vi "Analog Waveform DAQ Engine.vi"(8 "error in":errorcluster, 10 "DAQ Engine":refnum<notifier>, 11 "Sequence Context In":refnum<k7>) -> (0 "error out":errorcluster)   [LabVIEW 2023, in "LTT_TeststandSteptypes.lvlib"]
uses:
  LTT_TeststandSteptypes.lvlib
  HardwareAbstractionLayer_LVOOP/Main/Class Ref.ctl
  HardwareAbstractionLayer_LVOOP/DMM/DMM.lvclass
  HardwareAbstractionLayer_LVOOP/Function Generator/Function Generator.lvclass
  HardwareAbstractionLayer_LVOOP/Oscilloscope/Oscilloscope.lvclass
  HardwareAbstractionLayer_LVOOP/PowerSupply/PowerSupply.lvclass
  HardwareAbstractionLayer_LVOOP/Teststand/Teststand.lvclass
  HardwareAbstractionLayer_LVOOP/Analog Output/AO/AO.lvclass
  HardwareAbstractionLayer_LVOOP/Analog Input/AI/AI.lvclass
  HardwareAbstractionLayer_LVOOP/Database/Database.lvclass
  HardwareAbstractionLayer_LVOOP/Digital Output/DO_class/DO.lvclass
  HardwareAbstractionLayer_LVOOP/Digital Input/DI_class/DI.lvclass
  HardwareAbstractionLayer_LVOOP/PWM Output/PWM Output_class/PWM Output.lvclass
  HardwareAbstractionLayer_LVOOP/PWM Input/PWM Input_class/PWM Input.lvclass
  HardwareAbstractionLayer_LVOOP/NI Switch/NISwitch_class/NISwitch.lvclass
  HardwareAbstractionLayer_LVOOP/Modbus/Modbus_class/Modbus.lvclass
  HardwareAbstractionLayer_LVOOP/CAN/CAN Lib/CAN_class/CAN.lvclass
  HardwareAbstractionLayer_LVOOP/Main/Class Options.ctl
  <vilib>/Utility/error.llb/DialogType.ctl
  HardwareAbstractionLayer_LVOOP/Main/Main.lvclass
panel:
  in  "stop":bool
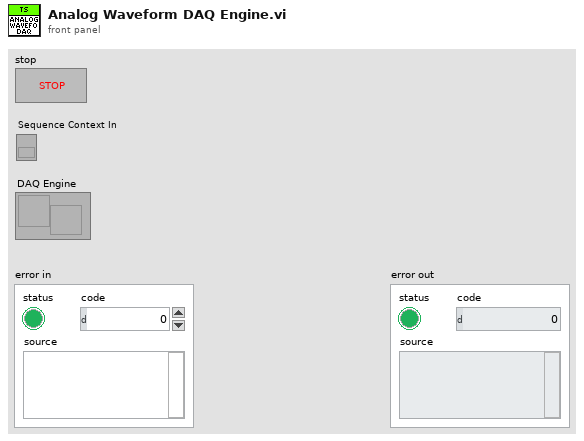
[diagram p1: front panel]
types:
  T1 = typedef "HardwareAbstractionLayer_LVOOP.lvlib/Main.lvclass/Class Ref.ctl" = cluster{"DMM":refnum<class "DMM.lvclass">, "Function Generator":refnum<class "Function Generator.lvclass">, "Oscilloscope":refnum<class "Oscilloscope.lvclass">, "PowerSupply":refnum<class "PowerSupply.lvclass">, "Teststand":refnum<class "Teststand.lvclass">, "AO":refnum<class "AO.lvclass">, "AI":refnum<class "AI.lvclass">, "Database":refnum<class "Database.lvclass">, "AO Waveform Generation":refnum<class "AO.lvclass">, "DO":refnum<class "DO.lvclass">, "DI":refnum<class "DI.lvclass">, "PWM Output":refnum<class "PWM Output.lvclass">, "PWM Input":refnum<class "PWM Input.lvclass">, "RelayOutput":refnum<class "NISwitch.lvclass">, "Modbus":refnum<class "Modbus.lvclass">, "CAN":refnum<class "CAN.lvclass">}
  T2 = typedef "HardwareAbstractionLayer_LVOOP.lvlib/Main.lvclass/Class Options.ctl" = enum16{"Init All Class", "Read All Class", "Write AI Class", "Write AO Class", "Write AO Waveform Generation", "Write DI Class", "Write DO Class", "Write PWM Input Class", "Write PWM Output Class", "Exit"}
  T3 = typedef "DialogType.ctl" = u16
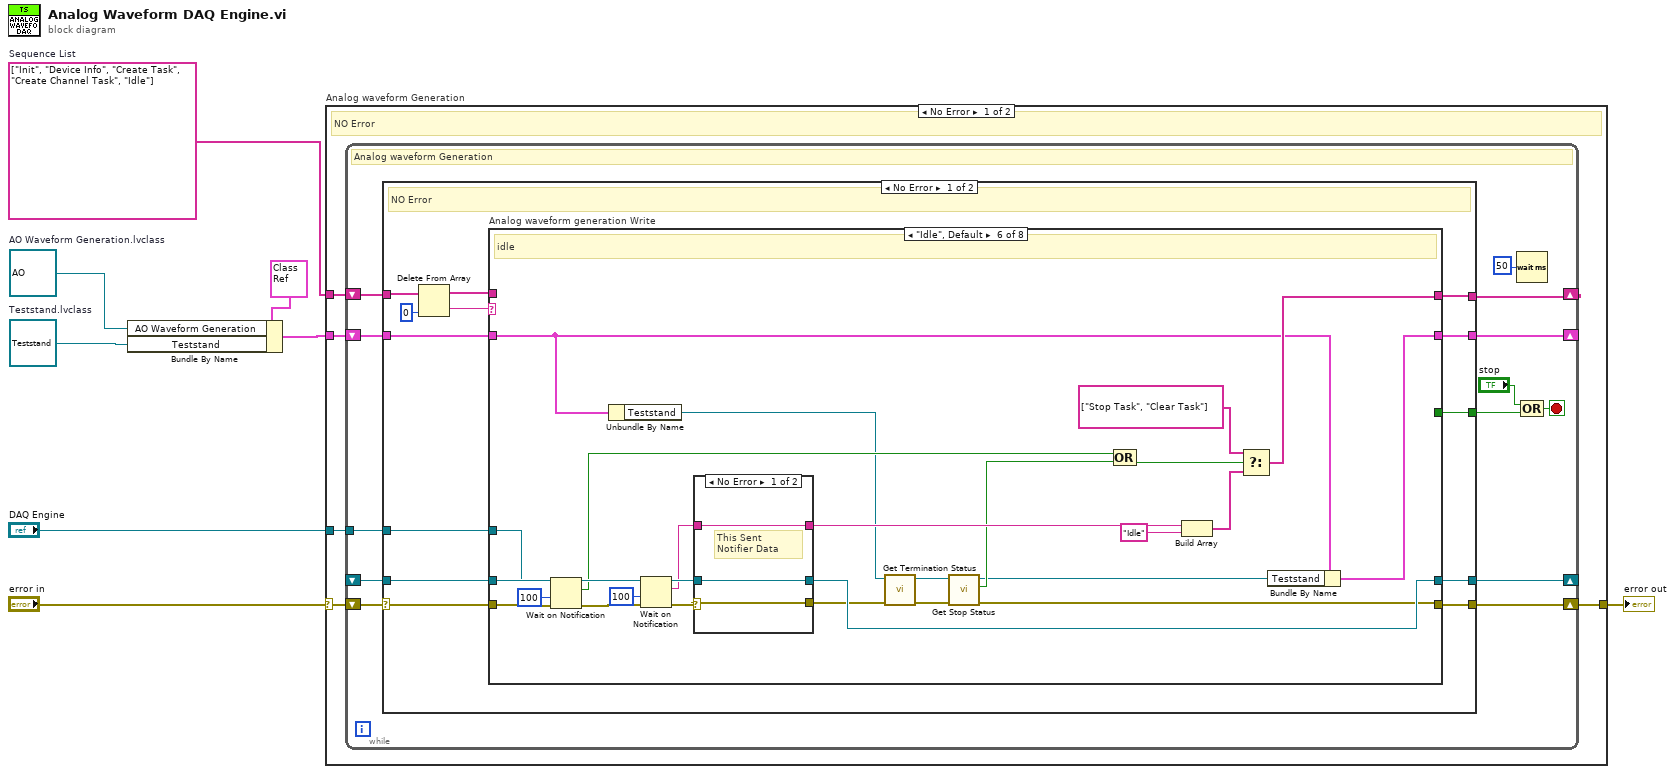
[diagram p0: block diagram]
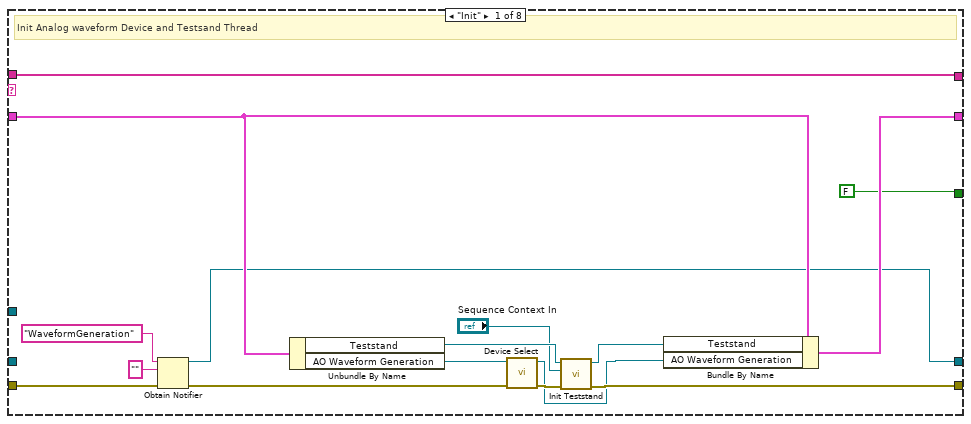
[diagram p2: hidden frame]
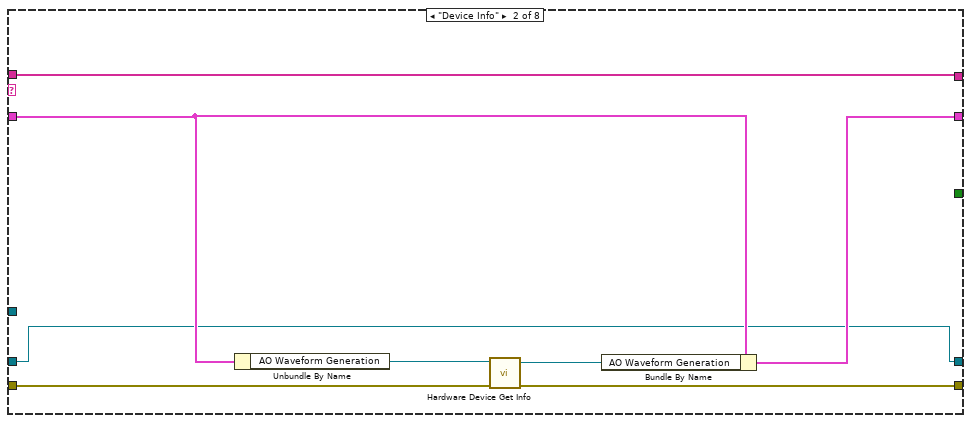
[diagram p3: hidden frame]
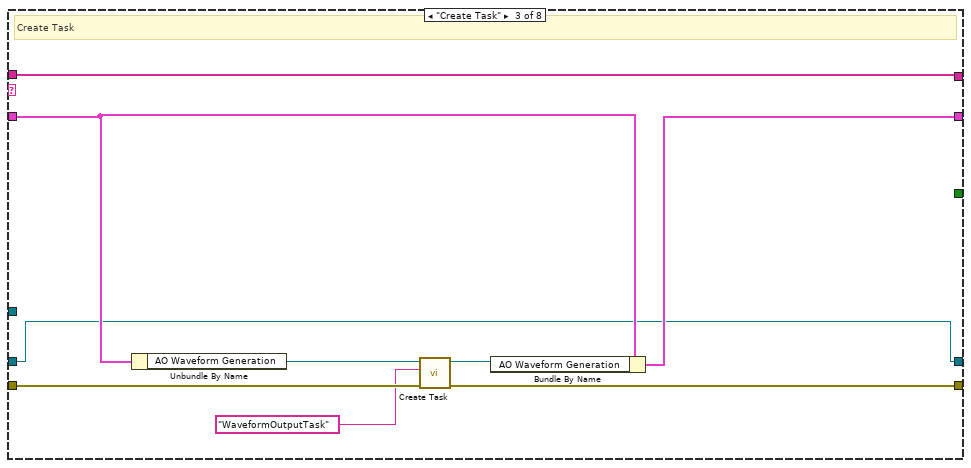
[diagram p4: hidden frame]
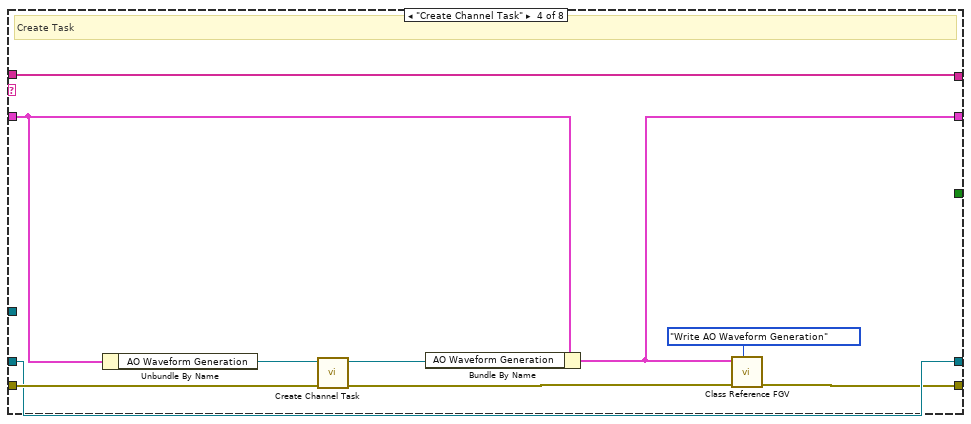
[diagram p5: hidden frame]
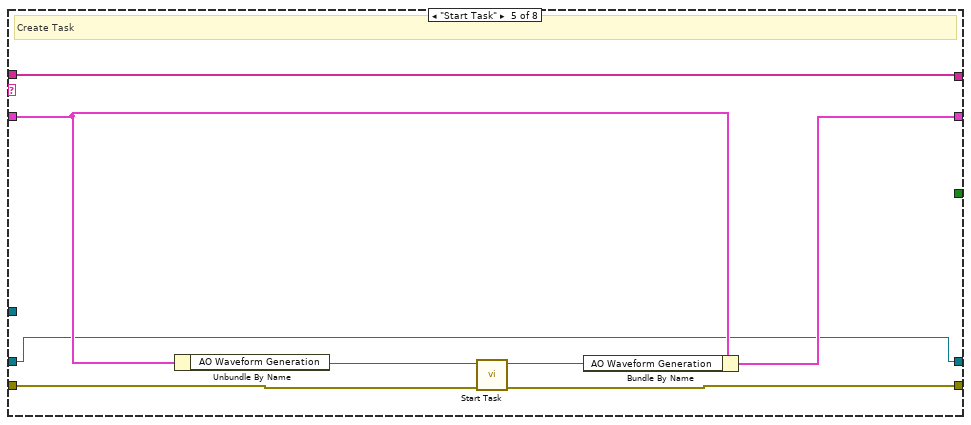
[diagram p6: hidden frame]
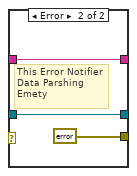
[diagram p7: hidden frame]
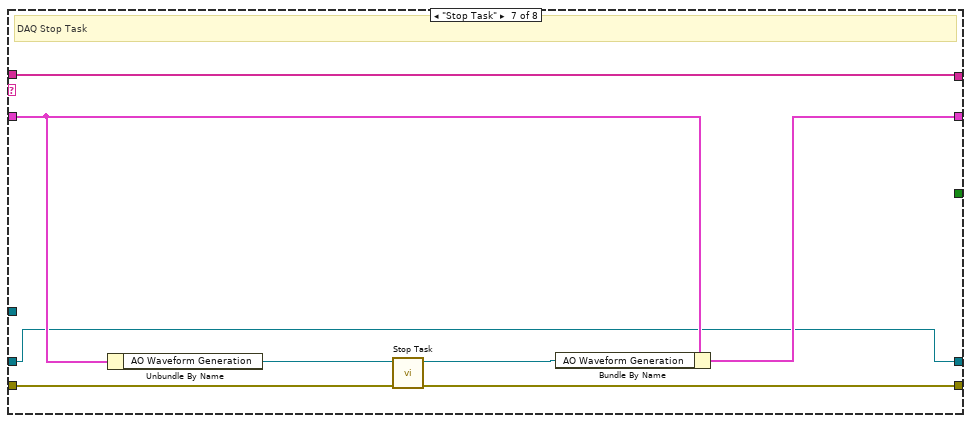
[diagram p8: hidden frame]
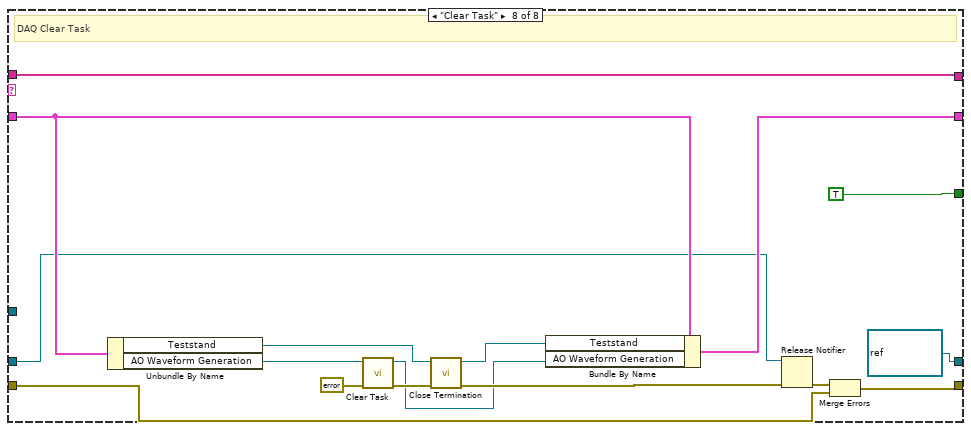
[diagram p9: hidden frame]
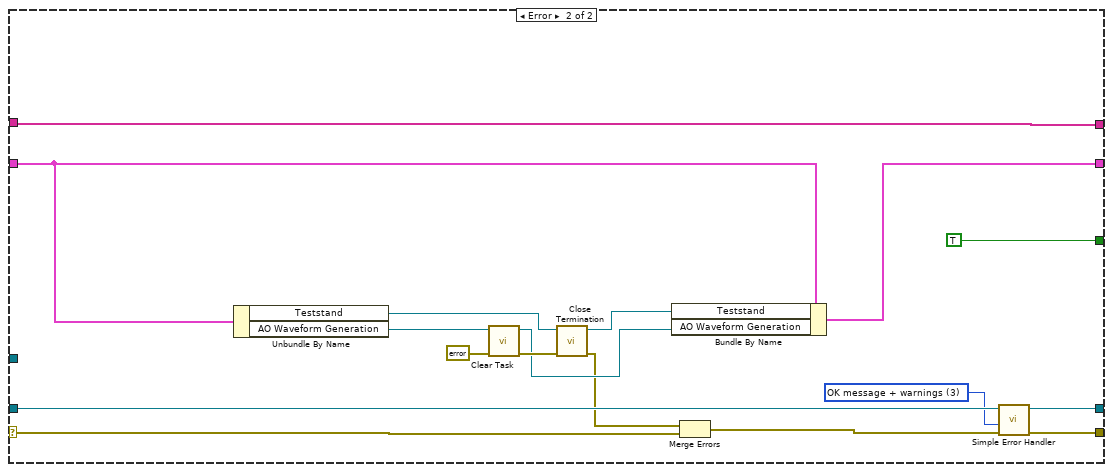
[diagram p10: hidden frame]
diagram:
  w1 = refnum<class "Teststand.lvclass"> refnum  # Teststand.lvclass
  w2 = refnum<class "AO.lvclass"> refnum  # AO Waveform Generation.lvclass
  w5 = string[] ["Init", "Device Info", "Create Task", "Create Channel Task", "Idle"]  # Sequence List
  n1 = Bundle By Name(cluster=T1 {"DMM"=refnum, "Function Generator"=refnum, "Oscilloscope"=refnum, "PowerSupply"=refnum, "Teststand"=refnum, "AO"=refnum, "AI"=refnum, "Database"=refnum, "AO Waveform Generation"=refnum, "DO"=refnum, "DI"=refnum, "PWM Output"=refnum, "PWM Input"=refnum, "RelayOutput"=refnum, "Modbus"=refnum, "CAN"=refnum} ("Class Cluster"), "AO Waveform Generation"=w2, "Teststand"=w1) -> (w6:T1)
  n2 = case "Analog waveform Generation" shown="No Error" "error in" {
    selector: "error in" -> [w13 w163]
    tunnel: [w12 w163] -> w8
    tunnel: w6 -> [w11 _]
    tunnel: w5 -> [w10 _]
    tunnel: "DAQ Engine" -> [w9 _]
    frame No Error {
      # "NO Error"
      n3 = while {
        shift-right: [w25] -> w12
        shift-left: w13 -> [w26]
        shift-right: [w23] -> _
        shift-left: w11 -> [w24]
        shift-right: [w21] -> _
        shift-left: w10 -> [w22]
        shift-right: [w16] -> _
        shift-left: _ -> [w15]
        tunnel: w9 -> [w14]
        stop <- w18 stop-if-true
        # "Analog waveform Generation"
        n4 = case shown="No Error" w26 {
          selector: w26 -> [w39 w160]
          tunnel: [w38 w148] -> w25
          tunnel: w24 -> [w34 w153]
          tunnel: [w33 w152] -> w23
          tunnel: w22 -> [w37 w150]
          tunnel: [w31 w150] -> w21
          tunnel: [w30 TRUE] -> w17
          tunnel: [w29 w161] -> w16
          tunnel: w15 -> [w28 w161]
          tunnel: w14 -> [w27 _]
          frame No Error {
            # "NO Error"
            n5 = Delete From Array(array=w37, index=0) -> (deleted portion=w36:string, array with subset deleted=w32:string[])  [unwired: 1 in]
            n6 = case "Analog waveform generation Write" shown="\"Idle\", Default" w36 {
              tunnel: w39 -> [w49 w60 w69 w80 w87 w104 w127 w132]
              tunnel: [w42 w59 w68 w75 w85 w92 w126 w133] -> w38
              tunnel: w34 -> [w54 w62 w71 w81 w89 w94 w129 w145]
              tunnel: [w53 w61 w70 w73 w88 w93 w128 w144] -> w33
              tunnel: w32 -> [w55 w63 w72 w82 w90 _ w130 w146]
              tunnel: [w55 w63 w72 w82 w90 w115 w130 w146] -> w31
              tunnel: [FALSE _ _ _ _ _ _ TRUE] -> w30
              tunnel: [w46 w56 w65 w77 w83 w108 w123 refnum<notifier> refnum ("notifier out")] -> w29
              tunnel: w28 -> [_ w56 w65 w77 w83 w113 w123 w141]
              tunnel: w27 -> [_ _ _ _ _ w102 _ _]
              frame "Init" {
                # "Init Analog waveform Device and Testsand Thread"
                n7 = Obtain Notifier(name (unnamed)="WaveformGeneration", notification data type="", error in (no error)=w49) -> (notifier out=w46:refnum<notifier>, error out=w48:errorcluster)  [unwired: 1 in, 1 out]
                n8 = Unbundle By Name(w54) -> ("Teststand"=w44:refnum<class "Teststand.lvclass">, "AO Waveform Generation"=w51:refnum<class "AO.lvclass">)
                n9 = call-dynamic "Device Select.vi"("error in (no error)"=w48, "AO in"=w51) -> ("error out"=w45:errorcluster, "AO out"=w41:refnum<class "AO.lvclass">)  [unwired: 8 in]
                n10 = call-dynamic "Init Teststand.vi"("error in (no error)"=w45, "Sequence Context In"="Sequence Context In", "Teststand in"=w44) -> ("error out"=w42:errorcluster, "Teststand out"=w43:refnum<class "Teststand.lvclass">)  [unwired: 7 in]
                n11 = Bundle By Name(cluster=w54, "Teststand"=w43, "AO Waveform Generation"=w41) -> (w53:T1)
              }
              frame "Device Info" {
                n12 = Unbundle By Name(w62) -> ("AO Waveform Generation"=w57:refnum<class "AO.lvclass">)
                n13 = call-dynamic "Hardware Device Get Info.vi"("error in (no error)"=w60, "AO in"=w57) -> ("error out"=w59:errorcluster, "AO out"=w58:refnum<class "AO.lvclass">)  [unwired: 8 in]
                n14 = Bundle By Name(cluster=w62, "AO Waveform Generation"=w58) -> (w61:T1)
              }
              frame "Create Task" {
                # "Create Task"
                n15 = Unbundle By Name(w71) -> ("AO Waveform Generation"=w66:refnum<class "AO.lvclass">)
                n16 = call-dynamic "Create Task.vi"("error in (no error)"=w69, "Task name"="WaveformOutputTask", "AO in"=w66) -> ("error out"=w68:errorcluster, "AO out"=w67:refnum<class "AO.lvclass">)  [unwired: 7 in]
                n17 = Bundle By Name(cluster=w71, "AO Waveform Generation"=w67) -> (w70:T1)
              }
              frame "Create Channel Task" {
                # "Create Task"
                n18 = Unbundle By Name(w81) -> ("AO Waveform Generation"=w78:refnum<class "AO.lvclass">)
                n19 = call-dynamic "Create Channel Task.vi"("error in (no error)"=w80, "AO in"=w78) -> ("error out"=w76:errorcluster, "AO out"=w79:refnum<class "AO.lvclass">)  [unwired: 8 in]
                n20 = Bundle By Name(cluster=w81, "AO Waveform Generation"=w79) -> (w73:T1)
                n21 = call "Class Reference FGV.vi"("Options"=Class_Options."Write AO Waveform Generation", "error in"=w76, "Class Cluster In"=w73) -> ("error out"=w75:errorcluster)  [unwired: 7 in, 1 out]
              }
              frame "Start Task" {
                # "Create Task"
                n22 = Unbundle By Name(w89) -> ("AO Waveform Generation"=w86:refnum<class "AO.lvclass">)
                n23 = call-dynamic "Start Task.vi"("error in (no error)"=w87, "AO in"=w86) -> ("error out"=w85:errorcluster, "AO out"=w84:refnum<class "AO.lvclass">)  [unwired: 8 in]
                n24 = Bundle By Name(cluster=w89, "AO Waveform Generation"=w84) -> (w88:T1)
              }
              frame "Idle", Default {
                # "idle"
                n25 = Wait on Notification(notifier=w102, timeout in ms (-1)=100, error in (no error)=w104) -> (notification=w100:bool, error out=w103:errorcluster)  [unwired: 1 in, 2 out]
                n26 = Unbundle By Name(w94) -> ("Teststand"=w99:refnum<class "Teststand.lvclass">)
                n27 = Wait on Notification(notifier=w113, timeout in ms (-1)=100, error in (no error)=w103) -> (notifier out=w109:refnum<notifier>, notification=w107:string, error out=w110:errorcluster)  [unwired: 1 in, 1 out]
                n28 = case shown="No Error" w110 {
                  selector: w110 -> [w119 _]
                  tunnel: [w119 errorcluster {"status"=FALSE, "code"=0, "source"=""} ("error IO")] -> w97
                  tunnel: w109 -> [w118 w122]
                  tunnel: [w118 w122] -> w108
                  tunnel: [w117 w121] -> w106
                  tunnel: w107 -> [w117 w121]
                  frame No Error {
                    # "This Sent Notifier Data"
                  }
                  frame Error {
                    # "This Error Notifier Data Parshing Emety"
                  }
                }
                n29 = call-dynamic "Get Termination Status.vi"("error in (no error)"=w97, "Teststand in"=w99) -> ("error out"=w96:errorcluster, "Teststand out"=w98:refnum<class "Teststand.lvclass">)  [unwired: 7 in, 1 out]
                n30 = call-dynamic "Get Stop Status.vi"("error in (no error)"=w96, "Teststand in"=w98) -> ("error out"=w92:errorcluster, "Value"=w95:bool, "Teststand out"=w91:refnum<class "Teststand.lvclass">)  [unwired: 7 in]
                n31 = Compound Arithmetic op=OR(w100, w95) -> (w114:bool)
                n32 = Build Array(w106, "Idle" ("element")) -> (w111:string[])
                n33 = Select(t=string[] ["Stop Task", "Clear Task"], s=w114, f=w111) -> (s? t:f=w115:string[])
                n34 = Bundle By Name(cluster=w94, "Teststand"=w91) -> (w93:T1)
              }
              frame "Stop Task" {
                # "DAQ Stop Task"
                n35 = Unbundle By Name(w129) -> ("AO Waveform Generation"=w124:refnum<class "AO.lvclass">)
                n36 = call-dynamic "Stop Task.vi"("error in (no error)"=w127, "AO in"=w124) -> ("error out"=w126:errorcluster, "AO out"=w125:refnum<class "AO.lvclass">)  [unwired: 8 in]
                n37 = Bundle By Name(cluster=w129, "AO Waveform Generation"=w125) -> (w128:T1)
              }
              frame "Clear Task" {
                # "DAQ Clear Task"
                n38 = Unbundle By Name(w145) -> ("Teststand"=w139:refnum<class "Teststand.lvclass">, "AO Waveform Generation"=w142:refnum<class "AO.lvclass">)
                n39 = call-dynamic "Clear Task.vi"("error in (no error)"=errorcluster {"status"=FALSE, "code"=0, "source"=""}, "AO in"=w142) -> ("error out"=w137:errorcluster, "AO out"=w134:refnum<class "AO.lvclass">)  [unwired: 8 in]
                n40 = call-dynamic "Close Termination.vi"("error in (no error)"=w137, "Teststand in"=w139) -> ("error out"=w136:errorcluster, "Teststand out"=w138:refnum<class "Teststand.lvclass">)  [unwired: 8 in]
                n41 = Bundle By Name(cluster=w145, "Teststand"=w138, "AO Waveform Generation"=w134) -> (w144:T1)
                n42 = Release Notifier(notifier=w141, error in (no error)=w136) -> (error out=w135:errorcluster)  [unwired: 1 in, 2 out]
                n43 = Merge Errors(w135, w132) -> (w133:errorcluster)
              }
            }
          }
          frame Error {
            w147 = T3 3 items=["no dialog", "OK message", "continue or stop message", "OK message + warnings", "continue/stop + warnings"] ("type of dialog (OK msg:1)")
            n44 = Unbundle By Name(w153) -> ("Teststand"=w158:refnum<class "Teststand.lvclass">, "AO Waveform Generation"=w159:refnum<class "AO.lvclass">)
            n45 = call-dynamic "Clear Task.vi"("error in (no error)"=errorcluster {"status"=FALSE, "code"=0, "source"=""}, "AO in"=w159) -> ("error out"=w156:errorcluster, "AO out"=w155:refnum<class "AO.lvclass">)  [unwired: 8 in]
            n46 = call-dynamic "Close Termination.vi"("error in (no error)"=w156, "Teststand in"=w158) -> ("error out"=w151:errorcluster, "Teststand out"=w157:refnum<class "Teststand.lvclass">)  [unwired: 8 in]
            n47 = Bundle By Name(cluster=w153, "Teststand"=w157, "AO Waveform Generation"=w155) -> (w152:T1)
            n48 = Merge Errors(w151, w160) -> (w149:errorcluster)
            n49 = call <vilib>:"Simple Error Handler.vi"("type of dialog (OK msg:1)"=w147, "error in (no error)"=w149) -> ("error out"=w148:errorcluster)  [unwired: 3 in, 4 out]
          }
        }
        n50 = Wait (ms)(milliseconds to wait=u32 50) -> ()  [unwired: 1 out]
        n51 = Compound Arithmetic op=OR("stop", w17) -> (w18:bool)
      }
    }
    frame Error {
      # "Error"
    }
  }
  "error out" <- w8
